vi "Read.vi"(0 "System Interface in":refnum<class "System Interface.lvclass">, 11 "Error In":errorcluster) -> (4 "System Interface out":refnum<class "System Interface.lvclass">, 6 "Process Data":T1, 15 "Error Out":errorcluster)   [LabVIEW 2020, in "Optitrack.lvlib"]
uses:
  <vilib>/ADAS Record/CustomDataTypes/Optitrack/Optitrack.lvlib
  <vilib>/ADAS Record/CustomDataTypes/Optitrack/Process Data.ctl
  4520f411-daba-4182-bc35-841ea590f987.vi
  Projects/NI AzDO/Mercedes-MPIC-201077/Record_MPIC3/mercedes-record-mpic3-201077/software-record-plugins/labview-2020/src/shared/TypeDef-Optitrack-RigidBody.ctl
  Projects/NI AzDO/Mercedes-MPIC-201077/Record_MPIC3/mercedes-record-mpic3-201077/software-record-plugins/labview-2020/src/shared/TypeDef-Optitrack-MarkerPoint.ctl
  Projects/NI AzDO/Mercedes-MPIC-201077/Record_MPIC3/mercedes-record-mpic3-201077/software-record-plugins/labview-2020/src/shared/TypeDef-Optitrack-MarkerSet.ctl
  Projects/NI AzDO/Mercedes-MPIC-201077/Record_MPIC3/mercedes-record-mpic3-201077/software-record-plugins/labview-2020/src/shared/TypeDef-Optitrack-LabeledMarker.ctl
  Projects/NI AzDO/Mercedes-MPIC-201077/Record_MPIC3/mercedes-record-mpic3-201077/software-record-plugins/labview-2020/src/shared/TypeDef-Optitrack-TrackedData.ctl
  Projects/NI AzDO/Mercedes-MPIC-201077/Record_MPIC3/mercedes-record-mpic3-201077/software-record-plugins/labview-2020/src/shared/TypeDef-Optitrack-FrameData.ctl
  <vilib>/FlexLogger/SDK/PluginSDK.lvlibp/PEFClasses/SDK/System Interface/System Interface.lvclass
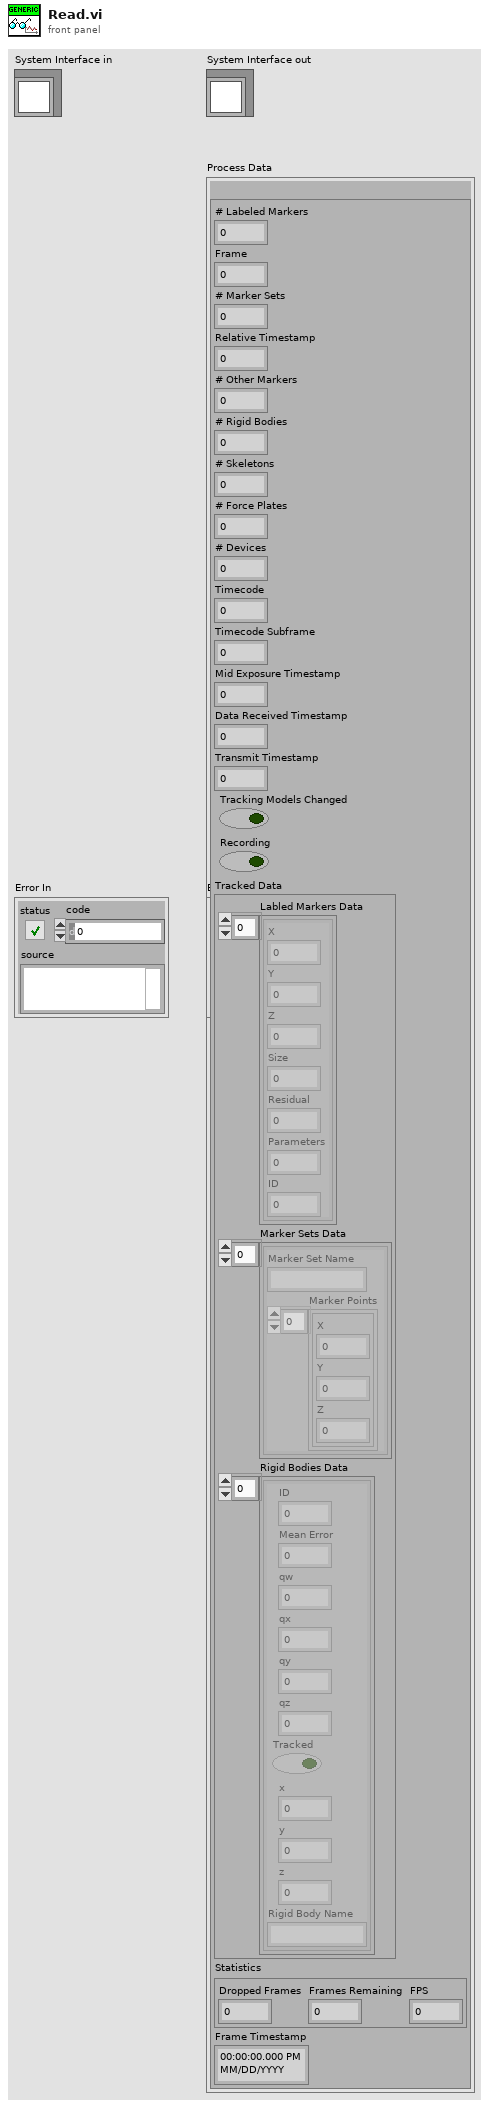
[diagram p1: front panel]
types:
  T1 = typedef "Optitrack.lvlib/Process Data.ctl" = cluster{"OptitrackFrame":T2}
  T2 = typedef "TypeDef-Optitrack-FrameData.ctl" = cluster{"# Labeled Markers":i32, "Frame":i32, "# Marker Sets":i32, "Relative Timestamp":dbl, "# Other Markers":i32, "# Rigid Bodies":i32, "# Skeletons":i32, "# Force Plates":i32, "# Devices":i32, "Timecode":u32, "Timecode Subframe":u32, "Mid Exposure Timestamp":u64, "Data Received Timestamp":u64, "Transmit Timestamp":u64, "Tracking Models Changed":bool, "Recording":bool, "Tracked Data":T3, "Statistics":cluster{"Dropped Frames":i32, "Frames Remaining":i32, "FPS":dbl}, "Frame Timestamp":timestamp}
  T3 = typedef "TypeDef-Optitrack-TrackedData.ctl" = cluster{"Labled Markers Data":T4[], "Marker Sets Data":T5[], "Rigid Bodies Data":T7[]}
  T4 = typedef "TypeDef-Optitrack-LabeledMarker.ctl" = cluster{"X":sgl, "Y":sgl, "Z":sgl, "Size":sgl, "Residual":sgl, "Parameters":i16, "ID":i32}
  T5 = typedef "TypeDef-Optitrack-MarkerSet.ctl" = cluster{"Marker Set Name":string, "Marker Points":T6[]}
  T6 = typedef "TypeDef-Optitrack-MarkerPoint.ctl" = cluster{"X":sgl, "Y":sgl, "Z":sgl}
  T7 = typedef "TypeDef-Optitrack-RigidBody.ctl" = cluster{"ID":i32, "Mean Error":sgl, "qw":sgl, "qx":sgl, "qy":sgl, "qz":sgl, "Tracked":bool, "x":sgl, "y":sgl, "z":sgl, "Rigid Body Name":string}
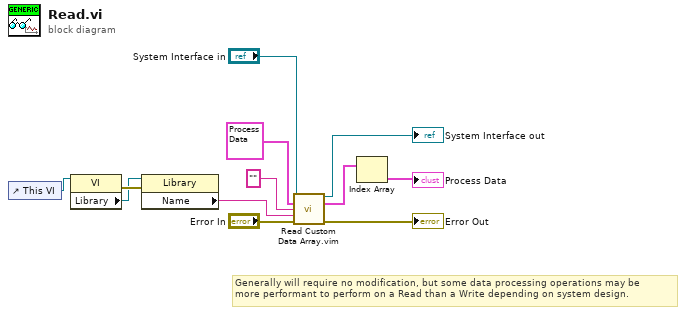
[diagram p0: block diagram]
diagram:
  # "Generally will require no modification, but some data processing operations may be\nmore performant to perform on a Read than a Write depending on system design."
  n1 = control-ref of="This VI"() -> (w4:refnum<vi>)
  n2 = property class="VI"(reference=w4) -> (error out=w3:errorcluster, "Library"=w2:refnum<vi>)  [unwired: 1 in, 1 out]
  n3 = property class="Library"(reference=w2, error in=w3) -> ("Name"=w1:string)  [unwired: 2 out]
  n4 = call "Read Custom Data Array.vim"("System Interface"="System Interface in", "Data Element Type"=T1 {"OptitrackFrame"={"# Labeled Markers"=0, "Frame"=0, "# Marker Sets"=0, "Relative Timestamp"=0.0, "# Other Markers"=0, "# Rigid Bodies"=0, "# Skeletons"=0, "# Force Plates"=0, "# Devices"=0, "Timecode"=0, "Timecode Subframe"=0, "Mid Exposure Timestamp"=0, "Data Received Timestamp"=0, "Transmit Timestamp"=0, "Tracking Models Changed"=FALSE, "Recording"=FALSE, "Tracked Data"={"Labled Markers Data"=[], "Marker Sets Data"=[], "Rigid Bodies Data"=[]}, "Statistics"={"Dropped Frames"=0, "Frames Remaining"=0, "FPS"=0.0}, "Frame Timestamp"=timestamp(0 s since 1904-01-01)}} ("Process Data"), "Metadata Element Type"="" ("appended array"), "Type"=w1, "error in (no error)"="Error In") -> ("System Interface out"=→"System Interface out":refnum<class "System Interface.lvclass">, "Data Array"=w5:T1[], "error out"=→"Error Out":errorcluster)  [unwired: 4 in, 4 out]
  n5 = Index Array(array=w5) -> (element=→"Process Data":T1)  [unwired: 1 in]
